vi "read_params.vi"(8 "error in (no error)":errorcluster, 11 "TweedieRegressor in":refnum<class "TweedieRegressor.lvclass">) -> (0 "error out":errorcluster, 2 "params":T1={"power"=0.0, "alpha"=1.0, "fit_intercept"=TRUE, "link"="auto", "max_iter"=100.0, "tol"=0.0001, "warm_start"=FALSE, "verbose"=0.0}, 3 "TweedieRegressor out":refnum<class "TweedieRegressor.lvclass">)   [LabVIEW 2020, in "TweedieRegressor.lvclass"]
uses:
  TweedieRegressor.lvclass
  Controls/tweedie_regressor_params.ctl
  TweedieRegressor.lvclass/TweedieRegressor.ctl
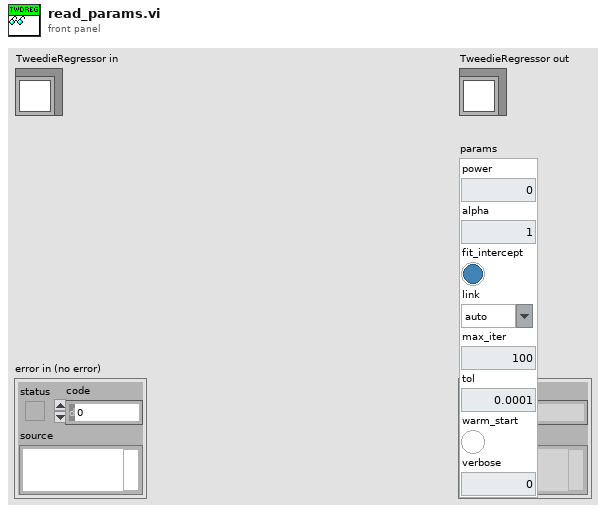
[diagram p1: front panel]
types:
  T1 = typedef "tweedie_regressor_params.ctl" = cluster{"power":dbl, "alpha":dbl, "fit_intercept":bool, "link":string, "max_iter":dbl, "tol":dbl, "warm_start":bool, "verbose":dbl}
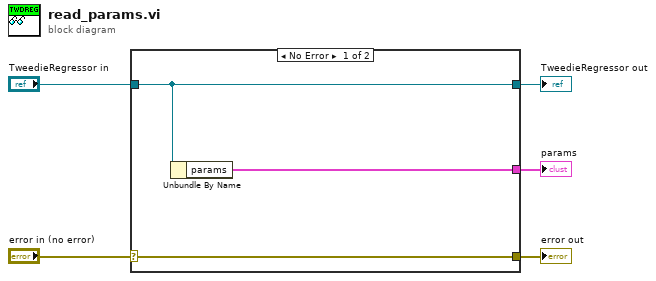
[diagram p0: block diagram]
diagram:
  n1 = case shown="No Error" "error in (no error)" {
    selector: "error in (no error)" -> [w8 w9]
    tunnel: [w8 w9] -> w4
    tunnel: [w7 w10] -> w2
    tunnel: "TweedieRegressor in" -> [w7 w10]
    tunnel: [w6 _] -> w1
    frame No Error {
      n2 = Unbundle By Name(w7) -> ("params"=w6:T1)
    }
    frame Error {
    }
  }
  "error out" <- w4
  "TweedieRegressor out" <- w2
  "params" <- w1
